vi "Camera Problem Fix.vi"(1 "Front Camera Modified":T1, 2 "Front Camera Original":T1) -> (0 "Front Camera Fixed":T1)   [LabVIEW 2013]
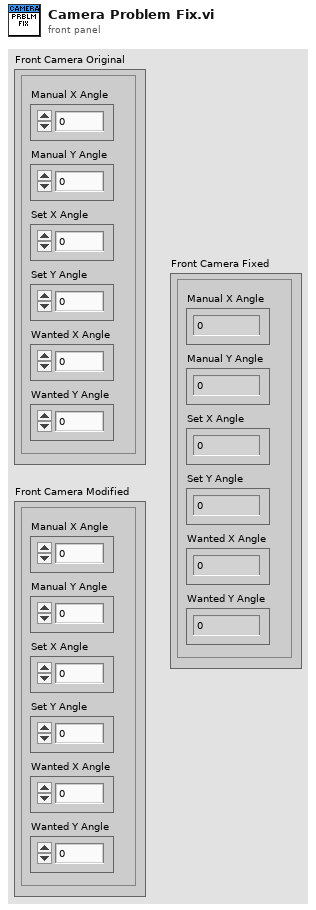
[diagram p1: front panel]
types:
  T1 = cluster{"Manual X Angle":dbl, "Manual Y Angle ":dbl, "Set X Angle":dbl, "Set Y Angle ":dbl, "Wanted X Angle":dbl, "Wanted Y Angle  ":dbl}
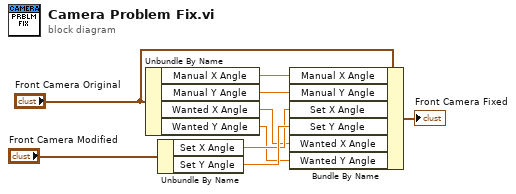
[diagram p0: block diagram]
diagram:
  n1 = Unbundle By Name("Front Camera Original") -> ("Manual X Angle"=w6:dbl, "Manual Y Angle"=w7:dbl, "Wanted X Angle"=w2:dbl, "Wanted Y Angle"=w1:dbl)
  n2 = Unbundle By Name("Front Camera Modified") -> ("Set X Angle"=w8:dbl, "Set Y Angle"=w9:dbl)
  n3 = Bundle By Name(cluster="Front Camera Original", "Manual X Angle"=w6, "Manual Y Angle"=w7, "Set X Angle"=w8, "Set Y Angle"=w9, "Wanted X Angle"=w2, "Wanted Y Angle"=w1) -> (→"Front Camera Fixed":T1)
